vi "Open PDF in desired reader.vi"(3 "Path":path) -> (0 "error out":errorcluster)   [LabVIEW 2020]
panel:
  out "Command string":string
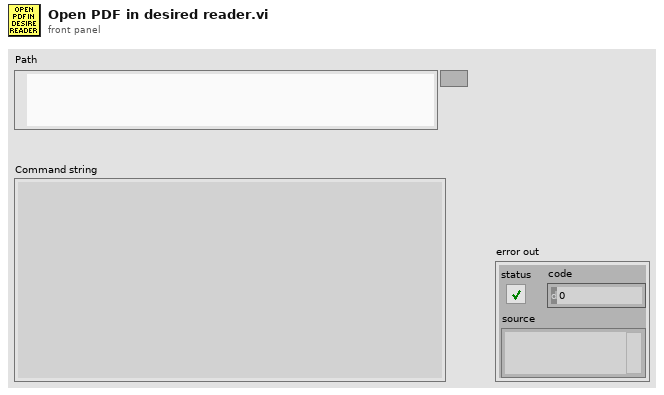
[diagram p1: front panel]
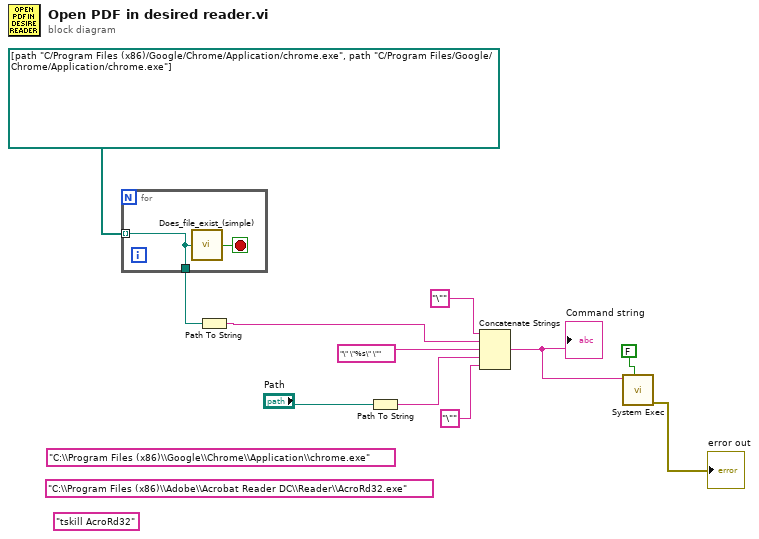
[diagram p0: block diagram]
diagram:
  (unwired) "C:\\Program Files (x86)\\Adobe\\Acrobat Reader DC\\Reader\\AcroRd32.exe"
  (unwired) "tskill AcroRd32"
  (unwired) "C:\\Program Files (x86)\\Google\\Chrome\\Application\\chrome.exe"
  n1 = for {
    tunnel: path[] [path "C:/Program Files (x86)/Google/Chrome/Application/chrome.exe", path "C:/Program Files/Google/Chrome/Application/chrome.exe"] -> [w12] mode=indexing
    tunnel: [w12] -> w5
    stop <- w13 stop-if-true
    n2 = call "Does_file_exist_(simple).vi"("Pathname"=w12) -> ("exists?"=w13:bool)
  }
  n3 = Path To String(path=w5) -> (string=w2:string)
  n4 = Path To String(path="Path") -> (string=w4:string)
  n5 = Concatenate Strings("\"" ("format string"), w2, "\" \"%s\" \"" ("format string"), w4, "\"" ("string")) -> (w8:string)
  "Command string" <- w8
  n6 = call <vilib>:"System Exec.vi"("wait until completion? (T)"=FALSE, "command line"=w8) -> ("error out"=→"error out":errorcluster)  [unwired: 6 in, 3 out]
